vi "主板信息配置.vi"(3 "从板个数":dbl=3.0, 5 "主板信息查看":string[][](table)=[["电池额定容量", "0"], ["电池实际容量", "0"], ["SOC", "0"], ["SOH", "0"], ["产品编号", ""], ["车架(牌)号", ""], ["配置文件版本", ""], ["从板1电池节数", "10"], ["从板2电池节数", "10"], ["从板3电池节数", "10"], ["从板1温度个数", "2"], ["从板2温度个数", "2"], ["从板3温度个数", "2"]]) -> (0 "输出数组":string[][](array[string]), 1 "布尔":bool, 2 "从板个数 2":dbl)   [LabVIEW 2013]
panel:
  in  "个数":string
  in  "个数":string
  in  "自动计算通道电压":bool
  in  "通道电压清零":bool
  in  "清空":bool
  in  "电压全设":bool
  in  "温度全设":bool
  in  "计算起始值":bool
  in  "停止":bool
  in  "确定":bool
  in  "项目信息":T1
  in  "保险位置":bool[][](array[boolean])
  in  "主板信息":string[][](table)
  in  "20个通道电压个数":u8[](array[numeric]) max=12
  # "主板保险位置最多支持10个"
  # "1"
  # "2"
  # "3"
  # "4"
  # "5"
  # "6"
  # "7"
  # "8"
  # "9"
  # "10"
  # "11"
  # "12"
  # "第一通道"
  # "第二通道"
  # "第三通道"
  # "第四通道"
  # "第五通道"
  # "第六通道"
  # "第七通道"
  # "第八通道"
  # "第九通道"
  # "第十通道"
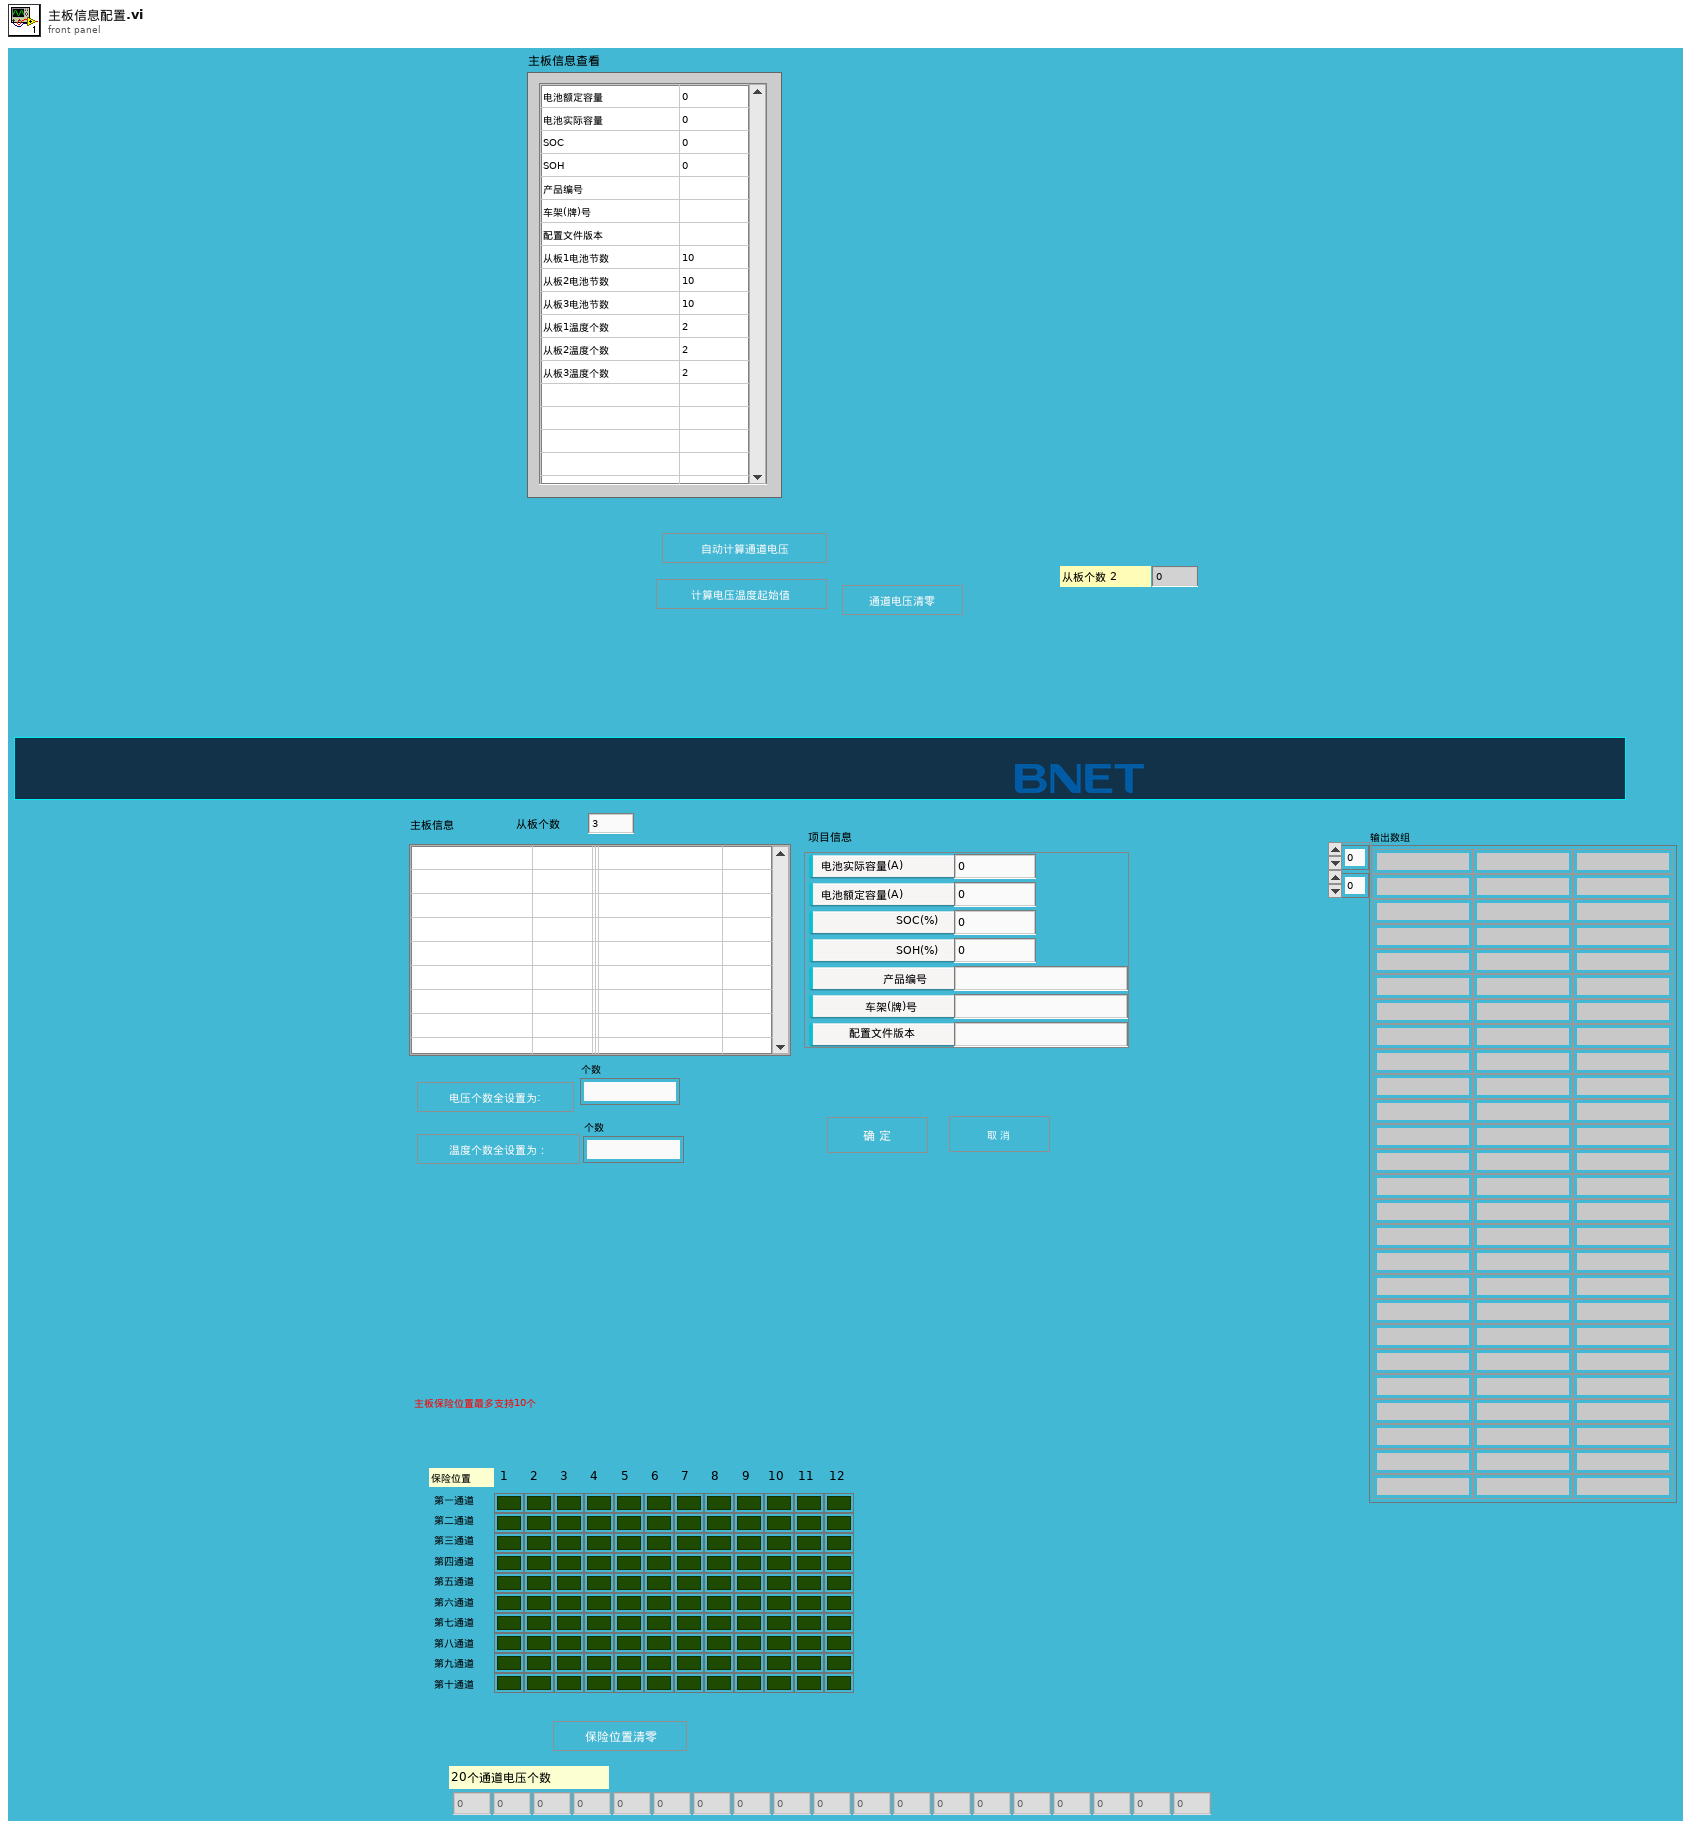
[diagram p1: front panel]
types:
  T1 = cluster{"电池额定容量(A)":dbl, "电池实际容量(A)":dbl, "SOC(%)":dbl, "SOH(%)":dbl, "产品编号":string, "车架(牌)号":string, "配置文件版本":string}
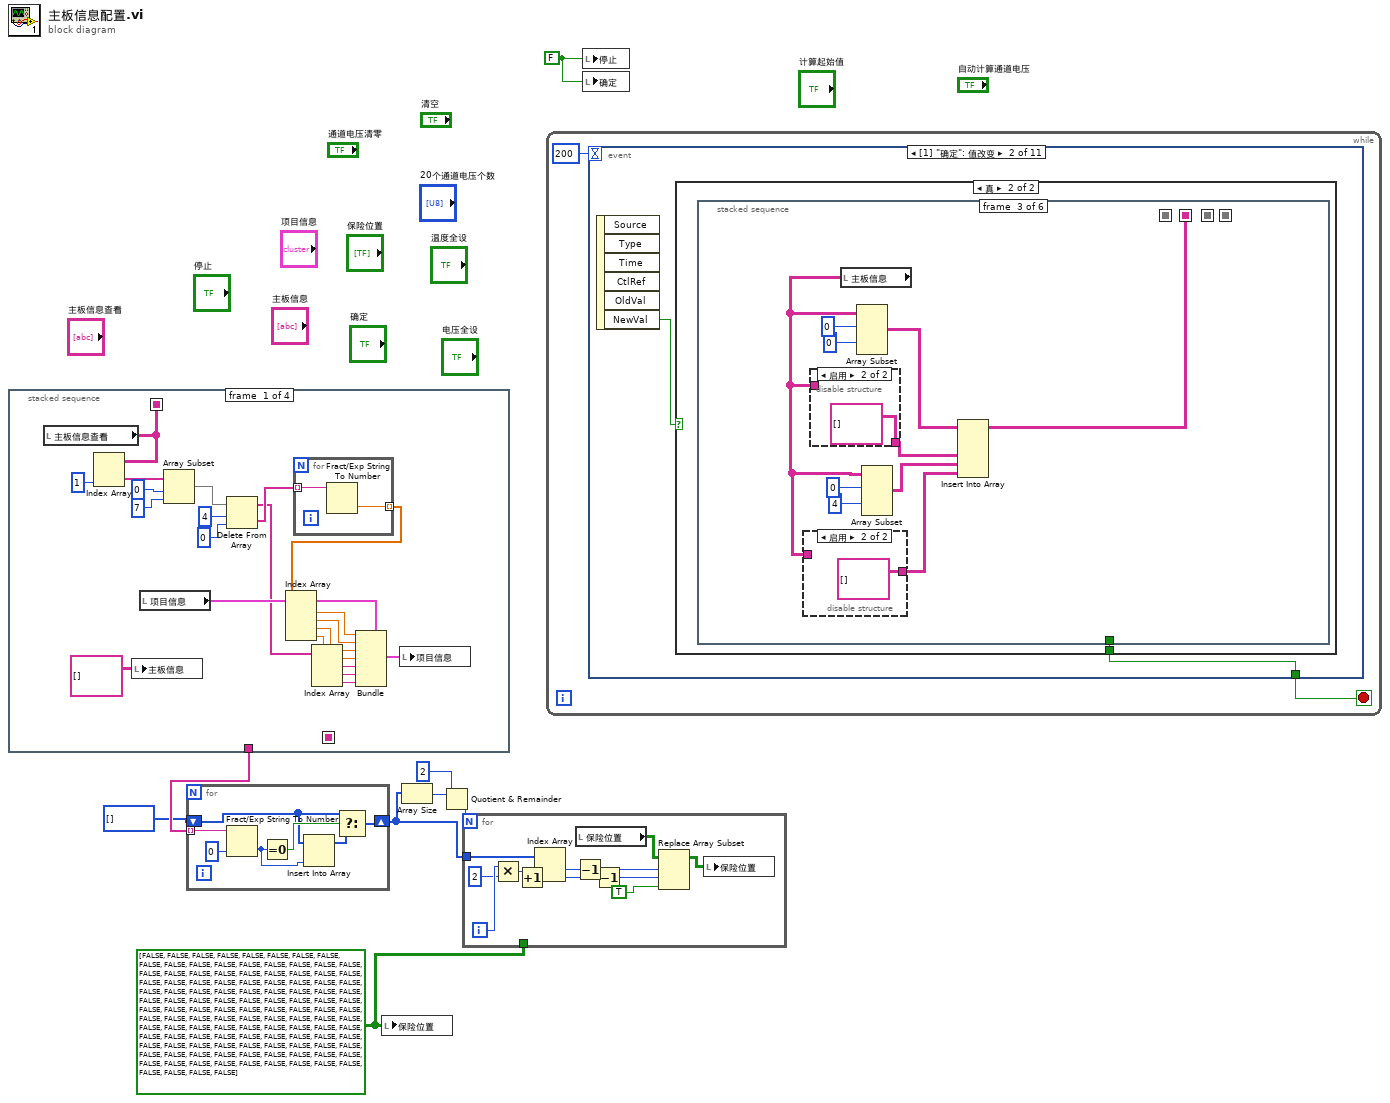
[diagram p0: block diagram]
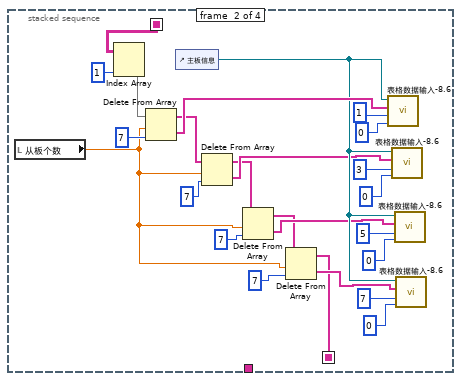
[diagram p2: hidden frame]
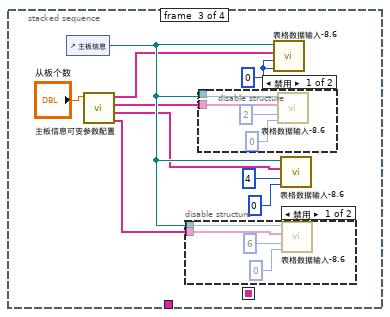
[diagram p3: hidden frame]
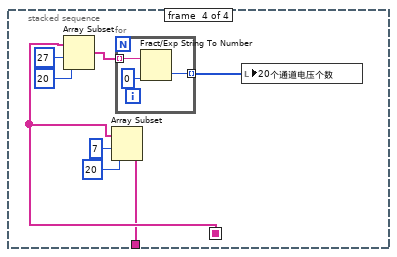
[diagram p6: hidden frame]
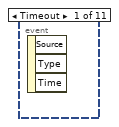
[diagram p7: hidden frame]
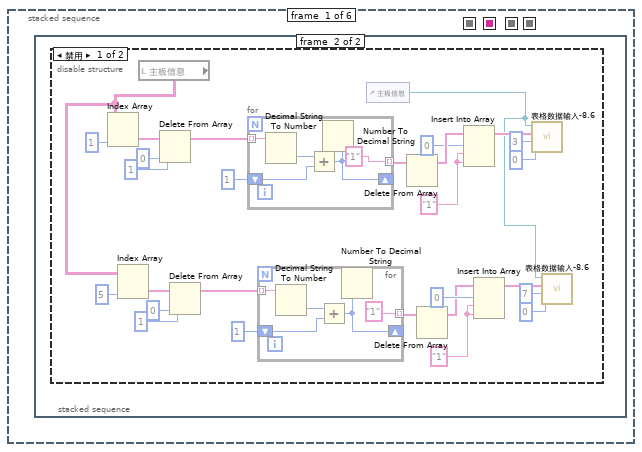
[diagram p9: hidden frame]
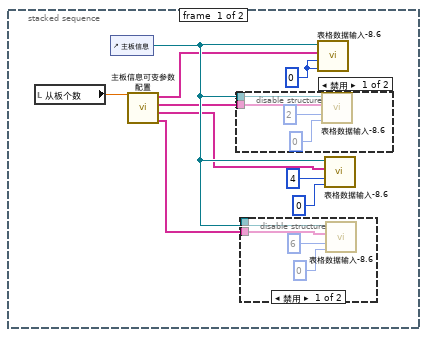
[diagram p10: hidden frame]
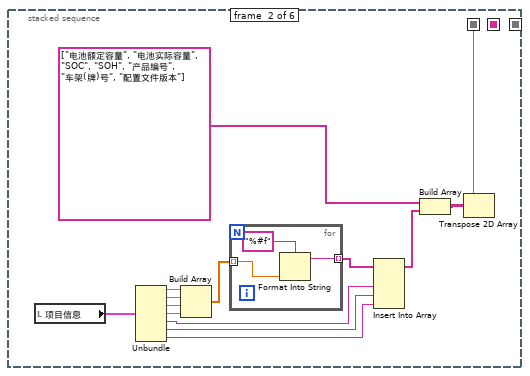
[diagram p14: hidden frame]
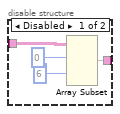
[diagram p15: hidden frame]
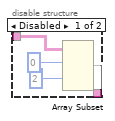
[diagram p16: hidden frame]
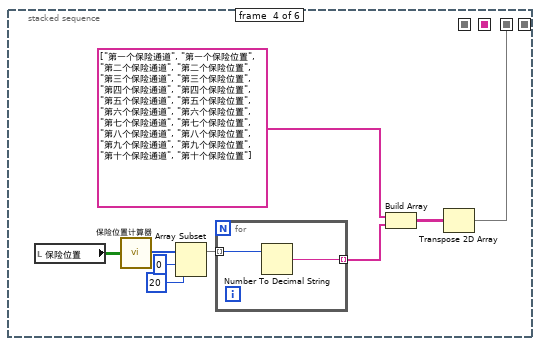
[diagram p17: hidden frame]
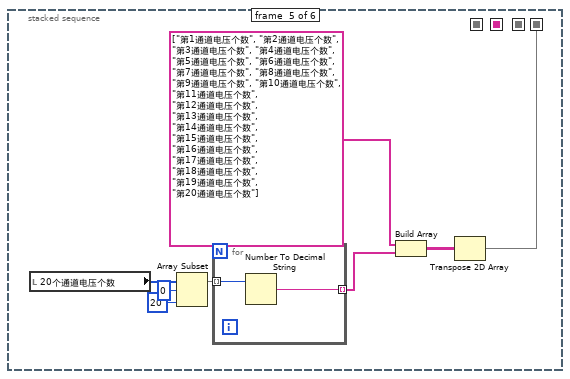
[diagram p18: hidden frame]
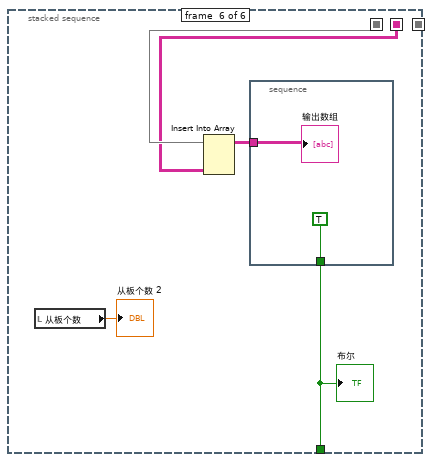
[diagram p19: hidden frame]
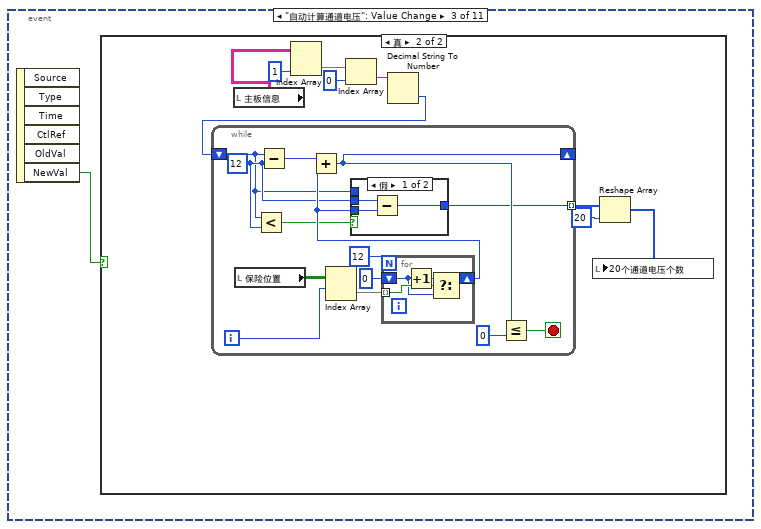
[diagram p20: hidden frame]
diagram:
  w2 = bool[][] [[FALSE, FALSE, FALSE, FALSE, FALSE, FALSE, FALSE, FALSE, FALSE, FALSE, FALSE, FALSE], [FALSE, FALSE, FALSE, FALSE, FALSE, FALSE, FALSE, FALSE, FALSE, FALSE, FALSE, FALSE], [FALSE, FALSE, FALSE, FALSE, FALSE, FALSE, FALSE, FALSE, FALSE, FALSE, FALSE, FALSE], [FALSE, FALSE, FALSE, FALSE, FALSE, FALSE, FALSE, FALSE, FALSE, FALSE, FALSE, FALSE], [FALSE, FALSE, FALSE, FALSE, FALSE, FALSE, FALSE, FALSE, FALSE, FALSE, FALSE, FALSE], [FALSE, FALSE, FALSE, FALSE, FALSE, FALSE, FALSE, FALSE, FALSE, FALSE, FALSE, FALSE], [FALSE, FALSE, FALSE, FALSE, FALSE, FALSE, FALSE, FALSE, FALSE, FALSE, FALSE, FALSE], [FALSE, FALSE, FALSE, FALSE, FALSE, FALSE, FALSE, FALSE, FALSE, FALSE, FALSE, FALSE], [FALSE, FALSE, FALSE, FALSE, FALSE, FALSE, FALSE, FALSE, FALSE, FALSE, FALSE, FALSE], [FALSE, FALSE, FALSE, FALSE, FALSE, FALSE, FALSE, FALSE, FALSE, FALSE, FALSE, FALSE]]
  w1 = FALSE ("取消按钮")
  n1 = stacked-sequence {
    seq-local: [w15 _ _ _] -> [_ w55 _ _]
    seq-local: [_ w33 _ _] -> [_ _ _ w75]
    tunnel: [_ _ _ w74] -> w8
    frame #0 {
      n2 = local read "主板信息查看"() -> (w15:string[][])
      n3 = Index Array(array=w15, index (col)=1 ("禁用的索引 (列)")) -> (element=w13:string[])  [unwired: 1 in]
      n4 = local write "主板信息"(string[][] [] ("主板信息")) -> ()
      n5 = local read "项目信息"() -> (w25:T1)
      n6 = Array Subset(array=w13, index=0 ("索引"), length=7 ("索引")) -> (w28:string[])
      n7 = Delete From Array(array=w28, length=4 ("长度"), index=0 ("索引 (行)")) -> (deleted portion=w26:string[], array with subset deleted=w10:string[])
      n8 = for {
        tunnel: w26 -> [w31] mode=indexing
        tunnel: [w30] -> w24 mode=indexing
        n9 = Fract/Exp String To Number(string=w31) -> (number=w30:dbl)  [unwired: 3 in, 1 out]
      }
      n10 = Index Array(array=w24) -> (element #1=w23:dbl, element #2=w22:dbl, element #3=w21:dbl, element #4=w20:dbl)  [unwired: 4 in]
      n11 = Index Array(array=w10) -> (element #1=w19:string, element #2=w18:string, element #3=w17:string)  [unwired: 3 in]
      n12 = Bundle(cluster=w25, "电池额定容量(A)"=w23, "电池实际容量(A)"=w22, "SOC(%)"=w21, "SOH(%)"=w20, "产品编号"=w19, "车架(牌)号"=w18, "配置文件版本"=w17) -> (w16:T1)
      n13 = local write "项目信息"(w16) -> ()
    }
    frame #1 {
      n14 = local read "从板个数"() -> (w32:dbl)
      n15 = Index Array(array=w55, index (col)=1 ("禁用的索引 (列)")) -> (element=w46:string[])  [unwired: 1 in]
      n16 = Delete From Array(array=w46, length=w32, index=7 ("索引")) -> (deleted portion=w44:string[], array with subset deleted=w42:string[])
      n17 = control-ref of="主板信息"() -> (w43:refnum<vi>)
      n18 = Delete From Array(array=w42, length=w32, index=7 ("索引")) -> (deleted portion=w40:string[], array with subset deleted=w39:string[])
      n19 = Delete From Array(array=w39, length=w32, index=7 ("索引")) -> (deleted portion=w37:string[], array with subset deleted=w36:string[])
      n20 = Delete From Array(array=w36, length=w32, index=7 ("索引")) -> (deleted portion=w34:string[], array with subset deleted=w33:string[])
      n21 = call "表格数据输入-8.6.vi"("行数"=u32 0, "列数"=u32 1 ("行数"), "字符串数组"=w44, "表格引用"=w43) -> ()  [unwired: 8 in]
      n22 = call "表格数据输入-8.6.vi"("行数"=u32 0, "列数"=u32 3 ("行数"), "字符串数组"=w40, "表格引用"=w43) -> ()  [unwired: 8 in]
      n23 = call "表格数据输入-8.6.vi"("行数"=u32 0, "列数"=u32 5 ("行数"), "字符串数组"=w37, "表格引用"=w43) -> ()  [unwired: 8 in]
      n24 = call "表格数据输入-8.6.vi"("行数"=u32 0, "列数"=u32 7 ("行数"), "字符串数组"=w34, "表格引用"=w43) -> ()  [unwired: 8 in]
    }
    frame #2 {
      w59 = u32 0 ("行数")
      n25 = control-ref of="主板信息"() -> (w65:refnum<vi>)
      n26 = call "主板信息可变参数配置.vi"("从板个数"="从板个数") -> ("主板温度起始值"=w64:string[], "主板温度个数"=w63:string[], "主板电压起始值"=w60:string[], "电池节数"=w58:string[])  [unwired: 7 in]
      n27 = disable-structure shown="禁用" {
        disable-tunnel: w65 -> [w69 _]
        disable-tunnel: w64 -> [w68 _]
        frame Disabled {
          n28 = call "表格数据输入-8.6.vi"("行数"=u32 0, "列数"=u32 6 ("行数"), "字符串数组"=w68, "表格引用"=w69) -> ()  [unwired: 8 in]
        }
        frame Enabled {
        }
      }
      n29 = disable-structure shown="禁用" {
        disable-tunnel: w65 -> [w73 _]
        disable-tunnel: w60 -> [w71 _]
        frame Disabled {
          n30 = call "表格数据输入-8.6.vi"("行数"=u32 0, "列数"=u32 2 ("行数"), "字符串数组"=w71, "表格引用"=w73) -> ()  [unwired: 8 in]
        }
        frame Enabled {
        }
      }
      n31 = call "表格数据输入-8.6.vi"("行数"=w59, "列数"=w59, "字符串数组"=w58, "表格引用"=w65) -> ()  [unwired: 8 in]
      n32 = call "表格数据输入-8.6.vi"("行数"=u32 0, "列数"=u32 4 ("行数"), "字符串数组"=w63, "表格引用"=w65) -> ()  [unwired: 8 in]
    }
    frame #3 {
      n33 = Array Subset(array=w75, index=27 ("索引"), length=20 ("索引")) -> (w80:string[])
      n34 = Array Subset(array=w75, index=7 ("索引"), length=20 ("索引")) -> (w74:string[])
      n35 = for {
        tunnel: w80 -> [w84] mode=indexing
        tunnel: [w83] -> w79 mode=indexing
        n36 = Fract/Exp String To Number(string=w84, default (0 dbl)=u8 0) -> (number=w83:u8)  [unwired: 2 in, 1 out]
      }
      n37 = local write "20个通道电压个数"(w79) -> ()
    }
  }
  n38 = for {
    tunnel: w8 -> [w91] mode=indexing
    shift-right: [w88] -> w4
    shift-left: i32[] [] -> [w87]
    n39 = Fract/Exp String To Number(string=w91, default (0 dbl)=u8 0) -> (number=w86:u8)  [unwired: 2 in, 1 out]
    n40 = Equal To 0?(x=w86) -> (x = 0?=w89:bool)
    n41 = Insert Into Array(array=w87, new element=w86) -> (w85:i32[])  [unwired: 1 in]
    n42 = Select(t=w87, s=w89, f=w85) -> (s? t:f=w88:i32[])
  }
  n43 = local write "保险位置"(w2) -> ()
  n44 = Array Size(array=w4) -> (size(s)=w6:i32)
  n45 = Quotient & Remainder(x=w6, y=2) -> (floor(x/y)=w3:i32)  [unwired: 1 out]
  n46 = for {
    N: w3 -> [_]
    tunnel: w4 -> [w103]
    tunnel: w2 -> [_]
    i -> [w102]
    n47 = Multiply(x=w102, y=2) -> (x*y=w100:i32)
    n48 = Increment(x=w100) -> (x+1=w99:i32)
    n49 = Index Array(array=w103, index #1=w100, index #2=w99) -> (element #1=w98:i32, element #2=w97:i32)
    n50 = Decrement(x=w98) -> (x-1=w95:i32)
    n51 = local read "保险位置"() -> (w93:bool[][])
    n52 = Decrement(x=w97) -> (x-1=w94:i32)
    n53 = Replace Array Subset(array=w93, new element=TRUE, index (row)=w95, index (col)=w94) -> (w92:bool[][])
    n54 = local write "保险位置"(w92) -> ()
  }
  n55 = while {
    stop <- w105 stop-if-true
    n56 = event shown="[1] \"确定\": 值改变" {
      selector: _ -> [_ _ _ _ _ _ _ _ _ _ _]
      dyn-events: _ -> [_ _ _ _ _ _ _ _ _ _ _]
      timeout: 200 -> [_ _ _ _ _ _ _ _ _ _ _]
      tunnel: [_ w106 _ _ _ _ _ _ _ w378 w383] -> w105
      event Timeout {
        n57 = event-data() -> ()  [unwired: 1 in, 3 out]
      }
      event "确定": Value Change {
        n58 = event-data() -> ("NewVal"=w107:bool)  [unwired: 1 in, 5 out]
        n59 = case shown="真" w107 {
          tunnel: [_ w108] -> w106
          frame False {
          }
          frame True {
            n60 = stacked-sequence {
              seq-local: [_ w164 _ _ _ _] -> [_ _ _ _ _ w226]
              seq-local: [_ _ w181 _ _ _] -> [_ _ _ _ _ w225]
              seq-local: [_ _ _ w204 _ _] -> [_ _ _ _ _ _]
              seq-local: [_ _ _ _ w215 _] -> [_ _ _ _ _ _]
              tunnel: [_ _ _ _ _ w223] -> w108
              frame #0 {
                n61 = stacked-sequence {
                  frame #0 {
                    w110 = u32 0 ("行数")
                    n62 = local read "从板个数"() -> (w117:dbl)
                    n63 = control-ref of="主板信息"() -> (w116:refnum<vi>)
                    n64 = call "主板信息可变参数配置.vi"("从板个数"=w117) -> ("主板温度起始值"=w115:string[], "主板温度个数"=w114:string[], "主板电压起始值"=w111:string[], "电池节数"=w109:string[])  [unwired: 7 in]
                    n65 = disable-structure shown="禁用" {
                      disable-tunnel: w116 -> [w125 _]
                      disable-tunnel: w111 -> [w123 _]
                      frame Disabled {
                        n66 = call "表格数据输入-8.6.vi"("行数"=u32 0, "列数"=u32 2 ("行数"), "字符串数组"=w123, "表格引用"=w125) -> ()  [unwired: 8 in]
                      }
                      frame Enabled {
                      }
                    }
                    n67 = disable-structure shown="禁用" {
                      disable-tunnel: w116 -> [w121 _]
                      disable-tunnel: w115 -> [w120 _]
                      frame Disabled {
                        n68 = call "表格数据输入-8.6.vi"("行数"=u32 0, "列数"=u32 6 ("行数"), "字符串数组"=w120, "表格引用"=w121) -> ()  [unwired: 8 in]
                      }
                      frame Enabled {
                      }
                    }
                    n69 = call "表格数据输入-8.6.vi"("行数"=w110, "列数"=w110, "字符串数组"=w109, "表格引用"=w116) -> ()  [unwired: 8 in]
                    n70 = call "表格数据输入-8.6.vi"("行数"=u32 0, "列数"=u32 4 ("行数"), "字符串数组"=w114, "表格引用"=w116) -> ()  [unwired: 8 in]
                  }
                  frame #1 {
                    n71 = disable-structure shown="禁用" {
                      frame Disabled {
                        w127 = "1"
                        w126 = "1"
                        n72 = local read "主板信息"() -> (w129:string[][])
                        n73 = Index Array(array=w129, index (col)=1 ("禁用的索引 (列)")) -> (element=w148:string[])  [unwired: 1 in]
                        n74 = Index Array(array=w129, index (col)=5 ("禁用的索引 (列)")) -> (element=w135:string[])  [unwired: 1 in]
                        n75 = Delete From Array(array=w148, length=1 ("长度"), index=0 ("索引")) -> (array with subset deleted=w147:string[])  [unwired: 1 out]
                        n76 = Delete From Array(array=w135, length=1 ("长度"), index=0 ("索引")) -> (array with subset deleted=w136:string[])  [unwired: 1 out]
                        n77 = for {
                          tunnel: w147 -> [w163] mode=indexing
                          shift-right: [w160] -> _
                          shift-left: 1 ("禁用的索引 (列)") -> [w161]
                          tunnel: ["1"] -> w152 mode=indexing
                          n78 = Decimal String To Number(string=w163) -> (number=w162:i32)  [unwired: 2 in, 1 out]
                          n79 = Add(x=w162, y=w161) -> (x+y=w160:i32)
                          n80 = Number To Decimal String(number=w160) -> ()  [unwired: 1 in, 1 out]
                        }
                        n81 = for {
                          tunnel: w136 -> [w158] mode=indexing
                          shift-right: [w155] -> _
                          shift-left: 1 ("禁用的索引 (列)") -> [w156]
                          tunnel: ["1"] -> w131 mode=indexing
                          n82 = Decimal String To Number(string=w158) -> (number=w157:i32)  [unwired: 2 in, 1 out]
                          n83 = Add(x=w157, y=w156) -> (x+y=w155:i32)
                          n84 = Number To Decimal String(number=w155) -> ()  [unwired: 1 in, 1 out]
                        }
                        n85 = control-ref of="主板信息"() -> (w128:refnum<vi>)
                        n86 = Delete From Array(array=w152) -> (array with subset deleted=w151:string[])  [unwired: 2 in, 1 out]
                        n87 = Delete From Array(array=w131) -> (array with subset deleted=w132:string[])  [unwired: 2 in, 1 out]
                        n88 = Insert Into Array(array=w151, index=0 ("索引"), new element #1=w126, new element #2=w126) -> (w144:string[])
                        n89 = Insert Into Array(array=w132, index=0 ("索引"), new element #1=w127, new element #2=w127) -> (w139:string[])
                        n90 = call "表格数据输入-8.6.vi"("行数"=u32 0, "列数"=u32 3, "字符串数组"=w144, "表格引用"=w128) -> ()  [unwired: 8 in]
                        n91 = call "表格数据输入-8.6.vi"("行数"=u32 0, "列数"=u32 7, "字符串数组"=w139, "表格引用"=w128) -> ()  [unwired: 8 in]
                      }
                      frame Enabled {
                      }
                    }
                  }
                }
              }
              frame #1 {
                n92 = local read "项目信息"() -> (w177:T1)
                n93 = Unbundle ("解除捆绑")(w177) -> ("电池额定容量(A)"=w175:dbl, "电池实际容量(A)"=w174:dbl, "SOC(%)"=w173:dbl, "SOH(%)"=w172:dbl, "产品编号"=w169:string, "车架(牌)号"=w168:string, "配置文件版本"=w167:string)
                n94 = Build Array(w175, w174, w173, w172) -> (w171:dbl[])
                n95 = for {
                  tunnel: w171 -> [w180] mode=indexing
                  tunnel: [w178] -> w170 mode=indexing
                  n96 = Format Into String(format string="%#f" ("格式字符串"), w180) -> (resulting string=w178:string)  [unwired: 2 in, 1 out]
                }
                n97 = Insert Into Array ("数组插入")(array=w170, new element #1=w169, new element #2=w168, new element #3=w167) -> (w166:string[])  [unwired: 1 in]
                n98 = Build Array ("创建数组")(string[] ["电池额定容量", "电池实际容量", "SOC", "SOH", "产品编号", "车架(牌)号", "配置文件版本"], w166) -> (w165:string[][])
                n99 = Transpose 2D Array ("二维数组转置")(2D array=w165) -> (transposed array=w164:string[][])
              }
              frame #2 {
                n100 = local read "主板信息"() -> (w186:string[][])
                n101 = disable-structure shown="启用" {
                  disable-tunnel: w186 -> [w192 _]
                  disable-tunnel: [w191 string[][] []] -> w182
                  frame Disabled {
                    n102 = Array Subset(array=w192, index (row)=0 ("索引"), index (col)=6 ("索引")) -> (w191:string[][])  [unwired: 2 in]
                  }
                  frame Enabled {
                  }
                }
                n103 = disable-structure shown="启用" {
                  disable-tunnel: w186 -> [w197 _]
                  disable-tunnel: [w196 string[][] []] -> w184
                  frame Disabled {
                    n104 = Array Subset(array=w197, index (row)=0 ("索引"), index (col)=2 ("索引")) -> (w196:string[][])  [unwired: 2 in]
                  }
                  frame Enabled {
                  }
                }
                n105 = Array Subset(array=w186, index (row)=0 ("索引"), index (col)=0 ("索引")) -> (w185:string[][])  [unwired: 2 in]
                n106 = Array Subset(array=w186, index (row)=0 ("索引"), index (col)=4 ("索引")) -> (w183:string[][])  [unwired: 2 in]
                n107 = Insert Into Array(array=w185, new element #1=w184, new element #2=w183, new element #3=w182) -> (w181:string[][])  [unwired: 2 in]
              }
              frame #3 {
                n108 = local read "保险位置"() -> (w209:bool[][])
                n109 = call "保险位置计算器.vi"("保险位置"=w209) -> ("输出数组"=w208:i32[])
                n110 = Array Subset(array=w208, index=0 ("索引"), length=20 ("长度")) -> (w203:i32[])
                n111 = for {
                  tunnel: w203 -> [w211] mode=indexing
                  tunnel: [w210] -> w207 mode=indexing
                  n112 = Number To Decimal String(number=w211) -> (decimal integer string=w210:string)  [unwired: 1 in]
                }
                n113 = Build Array(string[] ["第一个保险通道", "第一个保险位置", "第二个保险通道", "第二个保险位置", "第三个保险通道", "第三个保险位置", "第四个保险通道", "第四个保险位置", "第五个保险通道", "第五个保险位置", "第六个保险通道", "第六个保险位置", "第七个保险通道", "第七个保险位置", "第八个保险通道", "第八个保险位置", "第九个保险通道", "第九个保险位置", "第十个保险通道", "第十个保险位置"], w207) -> (w205:string[][])
                n114 = Transpose 2D Array(2D array=w205) -> (transposed array=w204:string[][])
              }
              frame #4 {
                n115 = local read "20个通道电压个数"() -> (w219:u8[])
                n116 = Array Subset(array=w219, index=0 ("索引"), length=20 ("长度")) -> (w214:u8[])
                n117 = for {
                  tunnel: w214 -> [w221] mode=indexing
                  tunnel: [w220] -> w218 mode=indexing
                  n118 = Number To Decimal String(number=w221) -> (decimal integer string=w220:string)  [unwired: 1 in]
                }
                n119 = Build Array(string[] ["第1通道电压个数", "第2通道电压个数", "第3通道电压个数", "第4通道电压个数", "第5通道电压个数", "第6通道电压个数", "第7通道电压个数", "第8通道电压个数", "第9通道电压个数", "第10通道电压个数", "第11通道电压个数", "第12通道电压个数", "第13通道电压个数", "第14通道电压个数", "第15通道电压个数", "第16通道电压个数", "第17通道电压个数", "第18通道电压个数", "第19通道电压个数", "第20通道电压个数"], w218) -> (w216:string[][])
                n120 = Transpose 2D Array(2D array=w216) -> (transposed array=w215:string[][])
              }
              frame #5 {
                n121 = local read "从板个数"() -> (→"从板个数 2":dbl)
                n122 = Insert Into Array(array=w226, new element=w225) -> (w224:string[][])  [unwired: 2 in]
                n123 = stacked-sequence {
                  tunnel: w224 -> [w228]
                  tunnel: [TRUE] -> w223
                  frame #0 {
                    "输出数组" <- w228
                  }
                }
                "布尔" <- w223
              }
            }
          }
        }
      }
      event "自动计算通道电压": Value Change {
        n124 = event-data() -> ("NewVal"=w229:bool)  [unwired: 1 in, 5 out]
        n125 = case shown="真" w229 {
          frame False {
          }
          frame True {
            n126 = local read "主板信息"() -> (w231:string[][])
            n127 = Index Array(array=w231, index (col)=1 ("禁用的索引 (列)")) -> (element=w233:string[])  [unwired: 1 in]
            n128 = Index Array(array=w233, index=0 ("索引")) -> (element=w235:string)
            n129 = Decimal String To Number(string=w235) -> (number=w236:i32)  [unwired: 2 in, 1 out]
            n130 = while {
              shift-right: [w245] -> _
              shift-left: w236 -> [w239]
              tunnel: [w243] -> w237 mode=indexing
              i -> [w252]
              stop <- w246 stop-if-true
              w241 = 12 ("y")
              n131 = local read "保险位置"() -> (w242:bool[][])
              n132 = Less?(x=w239, y=w241) -> (x < y?=w240:bool)
              n133 = Subtract(x=w239, y=w241) -> (x-y=w248:i32)
              n134 = Index Array(array=w242, index (row)=w252) -> (element=w251:bool[])  [unwired: 1 in]
              n135 = for {
                N: 12 -> [_]
                tunnel: w251 -> [w261] mode=indexing
                shift-right: [w262] -> w244
                shift-left: 0 -> [w259]
                n136 = Increment(x=w259) -> (x+1=w260:i32)
                n137 = Select(t=w260, s=w261, f=w259) -> (s? t:f=w262:i32)
              }
              n138 = Add(x=w248, y=w244) -> (x+y=w245:i32)
              n139 = case shown="假" w240 {
                tunnel: w244 -> [w255 w258]
                tunnel: [w254 w256] -> w243
                tunnel: w241 -> [w253 _]
                tunnel: w239 -> [_ w257]
                frame False {
                  n140 = Subtract(x=w253, y=w255) -> (x-y=w254:i32)
                }
                frame True {
                  n141 = Subtract(x=w257, y=w258) -> (x-y=w256:i32)
                }
              }
              n142 = Less Or Equal?(x=w245, y=0) -> (x <= y?=w246:bool)
            }
            n143 = Reshape Array(w237, 20 ("维数大小")) -> (w230:i32[])
            n144 = local write "20个通道电压个数"(w230) -> ()
          }
        }
      }
      event "清空": Value Change {
        n145 = event-data() -> ("NewVal"=w263:bool)  [unwired: 1 in, 5 out]
        n146 = case shown="真" w263 {
          frame False {
          }
          frame True {
            n147 = local write "保险位置"(bool[][] []) -> ()
          }
        }
      }
      event "通道电压清零": Value Change {
        n148 = event-data() -> ("NewVal"=w265:bool)  [unwired: 1 in, 5 out]
        n149 = case shown="真" w265 {
          frame False {
          }
          frame True {
            n150 = local write "20个通道电压个数"(i32[] [0, 0, 0, 0, 0, 0, 0, 0, 0, 0, 0, 0, 0, 0, 0, 0, 0, 0, 0, 0, 0] ("20个通道电压个数")) -> ()
          }
        }
      }
      event "计算起始值": Value Change {
        n151 = event-data() -> ("NewVal"=w267:bool)  [unwired: 1 in, 5 out]
        n152 = case shown="真" w267 {
          frame False {
          }
          frame True {
            n153 = stacked-sequence {
              frame #0 {
                w269 = u32 0 ("行数")
                n154 = local read "从板个数"() -> (w280:dbl)
                n155 = control-ref of="主板信息"() -> (w279:refnum<vi>)
                n156 = call "主板信息可变参数配置.vi"("从板个数"=w280) -> ("主板温度起始值"=w278:string[], "主板温度个数"=w275:string[], "主板电压起始值"=w271:string[], "电池节数"=w268:string[])  [unwired: 7 in]
                n157 = call "表格数据输入-8.6.vi"("行数"=w269, "列数"=w269, "字符串数组"=w268, "表格引用"=w279) -> ()  [unwired: 8 in]
                n158 = call "表格数据输入-8.6.vi"("行数"=u32 0, "列数"=u32 2 ("行数"), "字符串数组"=w271, "表格引用"=w279) -> ()  [unwired: 8 in]
                n159 = call "表格数据输入-8.6.vi"("行数"=u32 0, "列数"=u32 4 ("行数"), "字符串数组"=w275, "表格引用"=w279) -> ()  [unwired: 8 in]
                n160 = call "表格数据输入-8.6.vi"("行数"=u32 0, "列数"=u32 6 ("行数"), "字符串数组"=w278, "表格引用"=w279) -> ()  [unwired: 8 in]
              }
              frame #1 {
                w282 = "1"
                w281 = "1"
                n161 = local read "主板信息"() -> (w284:string[][])
                n162 = Index Array(array=w284, index (col)=1 ("禁用的索引 (列)")) -> (element=w303:string[])  [unwired: 1 in]
                n163 = Index Array(array=w284, index (col)=5 ("禁用的索引 (列)")) -> (element=w290:string[])  [unwired: 1 in]
                n164 = Delete From Array(array=w303, length=1 ("长度"), index=0 ("索引")) -> (array with subset deleted=w302:string[])  [unwired: 1 out]
                n165 = Delete From Array(array=w290, length=1 ("长度"), index=0 ("索引")) -> (array with subset deleted=w291:string[])  [unwired: 1 out]
                n166 = for {
                  tunnel: w302 -> [w318] mode=indexing
                  shift-right: [w315] -> _
                  shift-left: 1 ("禁用的索引 (列)") -> [w316]
                  tunnel: ["1"] -> w307 mode=indexing
                  n167 = Decimal String To Number(string=w318) -> (number=w317:i32)  [unwired: 2 in, 1 out]
                  n168 = Add(x=w317, y=w316) -> (x+y=w315:i32)
                  n169 = Number To Decimal String(number=w315) -> ()  [unwired: 1 in, 1 out]
                }
                n170 = for {
                  tunnel: w291 -> [w313] mode=indexing
                  shift-right: [w310] -> _
                  shift-left: 1 ("禁用的索引 (列)") -> [w311]
                  tunnel: ["1"] -> w286 mode=indexing
                  n171 = Decimal String To Number(string=w313) -> (number=w312:i32)  [unwired: 2 in, 1 out]
                  n172 = Add(x=w312, y=w311) -> (x+y=w310:i32)
                  n173 = Number To Decimal String(number=w310) -> ()  [unwired: 1 in, 1 out]
                }
                n174 = control-ref of="主板信息"() -> (w283:refnum<vi>)
                n175 = Delete From Array(array=w307) -> (array with subset deleted=w306:string[])  [unwired: 2 in, 1 out]
                n176 = Delete From Array(array=w286) -> (array with subset deleted=w287:string[])  [unwired: 2 in, 1 out]
                n177 = Insert Into Array(array=w306, index=0 ("索引"), new element #1=w281, new element #2=w281) -> (w299:string[])
                n178 = Insert Into Array(array=w287, index=0 ("索引"), new element #1=w282, new element #2=w282) -> (w294:string[])
                n179 = call "表格数据输入-8.6.vi"("行数"=u32 0, "列数"=u32 3, "字符串数组"=w299, "表格引用"=w283) -> ()  [unwired: 8 in]
                n180 = call "表格数据输入-8.6.vi"("行数"=u32 0, "列数"=u32 7, "字符串数组"=w294, "表格引用"=w283) -> ()  [unwired: 8 in]
              }
            }
          }
        }
      }
      event "温度全设": Value Change {
        n181 = event-data() -> ("NewVal"=w319:bool)  [unwired: 1 in, 5 out]
        n182 = case shown="真" w319 {
          frame False {
          }
          frame True {
            n183 = case shown="真" TRUE {
              tunnel: "个数" -> [_ w325]
              frame False {
              }
              frame True {
                n184 = local read "从板个数"() -> (w326:dbl)
                n185 = for {
                  N: w326 -> [_]
                  tunnel: w325 -> [w338]
                  tunnel: [w338] -> w323 mode=indexing
                  tunnel: [w337] -> w324 mode=indexing
                  n186 = Decimal String To Number(string=w338) -> (number=w337:i32)  [unwired: 2 in, 1 out]
                }
                n187 = control-ref of="主板信息"() -> (w327:refnum<vi>)
                n188 = disable-structure shown="启用" {
                  disable-tunnel: w324 -> [w335 _]
                  disable-tunnel: w323 -> [w333 w336]
                  disable-tunnel: [w330 w336] -> w322
                  frame Disabled {
                    n189 = Add Array Elements(numeric array=w335) -> (sum=w334:i32)
                    n190 = Number To Decimal String(number=w334) -> (decimal integer string=w332:string)  [unwired: 1 in]
                    n191 = Insert Into Array(array=w333, index=0 ("索引"), new element=w332) -> (w330:string[])
                  }
                  frame Enabled {
                  }
                }
                n192 = call "表格数据输入-8.6.vi"("行数"=u32 0, "列数"=u32 5, "字符串数组"=w322, "表格引用"=w327) -> ()  [unwired: 8 in]
              }
            }
          }
        }
      }
      event "电压全设": Value Change {
        n193 = event-data() -> ("NewVal"=w339:bool)  [unwired: 1 in, 5 out]
        n194 = case shown="真" w339 {
          frame False {
          }
          frame True {
            n195 = case shown="真" TRUE {
              tunnel: "个数" -> [_ w345]
              frame False {
              }
              frame True {
                n196 = local read "从板个数"() -> (w346:dbl)
                n197 = for {
                  N: w346 -> [_]
                  tunnel: w345 -> [w358]
                  tunnel: [w358] -> w343 mode=indexing
                  tunnel: [w357] -> w344 mode=indexing
                  n198 = Decimal String To Number(string=w358) -> (number=w357:i32)  [unwired: 2 in, 1 out]
                }
                n199 = control-ref of="主板信息"() -> (w347:refnum<vi>)
                n200 = disable-structure shown="启用" {
                  disable-tunnel: w344 -> [w355 _]
                  disable-tunnel: w343 -> [w353 w356]
                  disable-tunnel: [w350 w356] -> w342
                  frame Disabled {
                    n201 = Add Array Elements(numeric array=w355) -> (sum=w354:i32)
                    n202 = Number To Decimal String(number=w354) -> (decimal integer string=w352:string)  [unwired: 1 in]
                    n203 = Insert Into Array(array=w353, index=0 ("索引"), new element=w352) -> (w350:string[])
                  }
                  frame Enabled {
                  }
                }
                n204 = call "表格数据输入-8.6.vi"("行数"=u32 0, "列数"=u32 1, "字符串数组"=w342, "表格引用"=w347) -> ()  [unwired: 8 in]
              }
            }
          }
        }
      }
      event "从板个数": Value Change {
        n205 = event-data() -> ("NewVal"=w359:dbl)  [unwired: 1 in, 5 out]
        n206 = stacked-sequence {
          tunnel: w359 -> [_ w369]
          frame #0 {
            n207 = local write "主板信息"(string[][] [] ("主板信息可变参数（根据从板个数多少变化）")) -> ()
          }
          frame #1 {
            w367 = u32 0 ("行数")
            n208 = control-ref of="主板信息"() -> (w361:refnum<vi>)
            n209 = call "主板信息可变参数配置.vi"("从板个数"=w369) -> ("主板温度起始值"=w362:string[], "主板温度个数"=w363:string[], "主板电压起始值"=w366:string[], "电池节数"=w368:string[])  [unwired: 7 in]
            n210 = disable-structure shown="禁用" {
              disable-tunnel: w366 -> [w372 _]
              disable-tunnel: w361 -> [w370 _]
              frame Disabled {
                n211 = call "表格数据输入-8.6.vi"("行数"=u32 0, "列数"=u32 2 ("行数"), "字符串数组"=w372, "表格引用"=w370) -> ()  [unwired: 8 in]
              }
              frame Enabled {
              }
            }
            n212 = disable-structure shown="禁用" {
              disable-tunnel: w362 -> [w375 _]
              disable-tunnel: w361 -> [w374 _]
              frame Disabled {
                n213 = call "表格数据输入-8.6.vi"("行数"=u32 0, "列数"=u32 6 ("行数"), "字符串数组"=w375, "表格引用"=w374) -> ()  [unwired: 8 in]
              }
              frame Enabled {
              }
            }
            n214 = call "表格数据输入-8.6.vi"("行数"=w367, "列数"=w367, "字符串数组"=w368, "表格引用"=w361) -> ()  [unwired: 8 in]
            n215 = call "表格数据输入-8.6.vi"("行数"=u32 0, "列数"=u32 4 ("行数"), "字符串数组"=w363, "表格引用"=w361) -> ()  [unwired: 8 in]
          }
        }
      }
      event "停止": Value Change {
        n216 = event-data() -> ()  [unwired: 1 in, 6 out]
        n217 = stacked-sequence {
          tunnel: [TRUE] -> w378
          frame #0 {
            n218 = local write "输出数组"(string[][] [] ("输出数组")) -> ()
            n219 = local write "布尔"(FALSE ("布尔")) -> ()
          }
        }
      }
      event Panel Close? {
        n220 = event-data() -> ()  [unwired: 1 in, 4 out]
        n221 = stacked-sequence {
          tunnel: [TRUE] -> w383
          frame #0 {
            n222 = local write "输出数组"(string[][] [] ("输出数组")) -> ()
            n223 = local write "布尔"(FALSE ("布尔")) -> ()
          }
        }
        n224 = event-data("Discard?"=FALSE ("放弃？")) -> ()  [unwired: 1 in, 1 out]
      }
    }
  }
  n225 = local write "停止"(w1) -> ()
  n226 = local write "确定"(w1) -> ()
